vi "pomocniczy.vi"() -> ()   [LabVIEW 2020]
panel:
  out "refnum out":refnum<file>
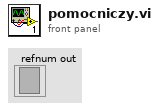
[diagram p1: front panel]
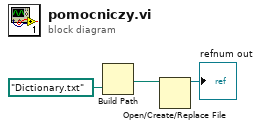
[diagram p0: block diagram]
diagram:
  n1 = Build Path(name or relative path=path "Dictionary.txt") -> (appended path=w2:path)  [unwired: 1 in]
  n2 = Open/Create/Replace File(file path (use dialog)=w2) -> (refnum out=→"refnum out":refnum<file>)  [unwired: 5 in, 2 out]
